vi "Stamp Version.vi"(8 "error in (no error)":errorcluster, 11 "Serial port":refnum<visa-resource-name>) -> (0 "error out":errorcluster, 1 "success":bool, 2 "version":string, 3 "Serial port out":refnum<visa-resource-name>)   [LabVIEW 2012]
panel:
  out "x-y":u32
  in  "versions":string="AB"
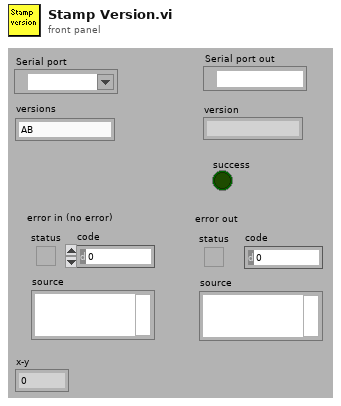
[diagram p1: front panel]
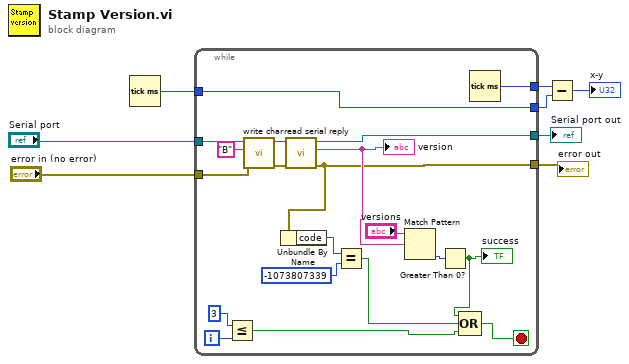
[diagram p0: block diagram]
diagram:
  n1 = Tick Count (ms)() -> (millisecond timer value=w2:u32)
  n2 = while {
    tunnel: [w27] -> w8
    tunnel: "Serial port" -> [w26]
    tunnel: [w13] -> w6
    tunnel: "error in (no error)" -> [w20]
    tunnel: [w15] -> w4
    tunnel: [w14] -> w3
    tunnel: w2 -> [w14]
    i -> [w19]
    stop <- w16 stop-if-true
    n3 = Less Or Equal?(x=3, y=w19) -> (x <= y?=w17:bool)
    n4 = call "write char.vi"("error in (no error)"=w20, "write buffer"="B", "Serial port"=w26) -> ("error out"=w24:errorcluster, "Serial Port"=w28:refnum<visa-resource-name>)  [unwired: 6 in, 1 out]
    n5 = call "read serial reply.vi"("error in (no error)"=w24, "Serial Port"=w28) -> ("error out"=w13:errorcluster, "reply"=w22:string, "Serial Port out"=w27:refnum<visa-resource-name>)  [unwired: 7 in]
    "version" <- w22
    n6 = Unbundle By Name(w13) -> ("code"=w11:i32)
    n7 = Equal?(x=w11, y=-1073807339) -> (x = y?=w9:bool)
    n8 = Match Pattern(string="versions", regular expression=w22) -> (offset past match=w21:i32)  [unwired: 1 in, 3 out]
    n9 = Greater Than 0?(x=w21) -> (x > 0?=w12:bool)
    "success" <- w12
    n10 = Compound Arithmetic op=OR(w12, w9, w17) -> (w16:bool)
    n11 = Tick Count (ms)() -> (millisecond timer value=w15:u32)
  }
  "Serial port out" <- w8
  "error out" <- w6
  n12 = Subtract(x=w4, y=w3) -> (x-y=→"x-y":u32)
